vi "Display Raw Data.vi"(6 "Display":T2=enum."Channel B", 7 "Enum":T1, 8 "Data Format":T3, 9 "Processed B-Scan":sgl[][](array[numeric]), 10 "Length":i32, 11 "Raw Data In":u16[](array[numeric])) -> ()   [LabVIEW 2014]
uses:
  Type Defs/OCT DAQ Channel Data Type.ctl
  Type Defs/Display States.ctl
  Display Raw Data states.ctl
panel:
  out "Raw Data":u16[](graph)
  out "FFT Data":sgl[](graph)
  in  "Index":i32
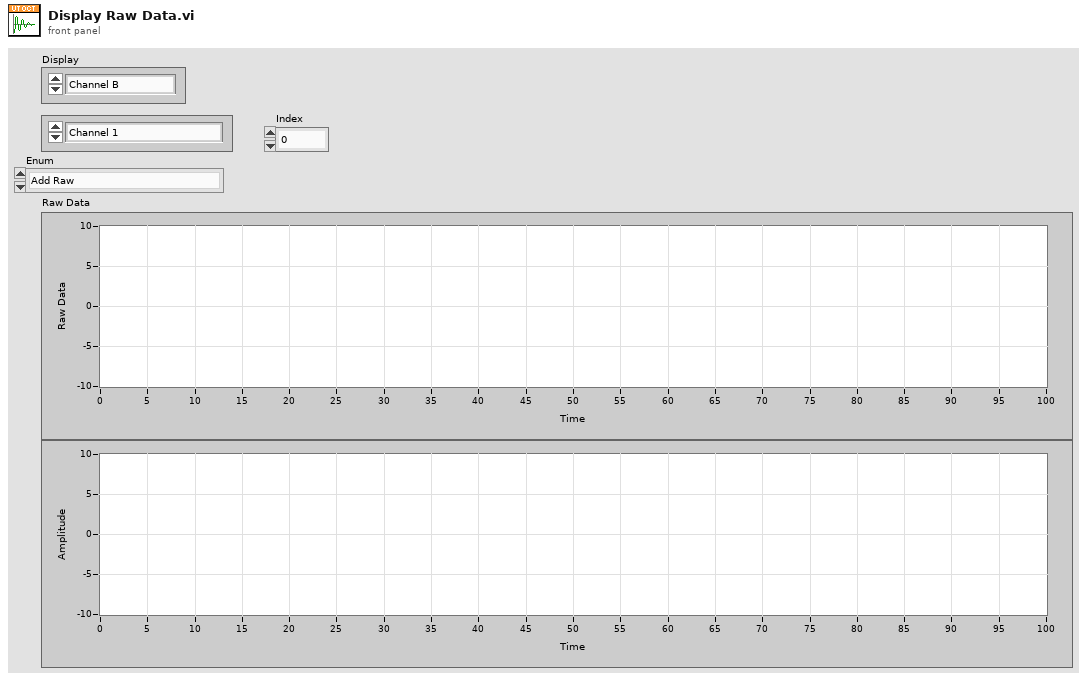
[diagram p1: front panel]
types:
  T1 = typedef "Display Raw Data states.ctl" = enum16{"Add Raw", "Add Processed", "Show"}
  T2 = typedef "Display States.ctl" = enum16{"Channel A", "Channel B"}
  T3 = typedef "OCT DAQ Channel Data Type.ctl" = enum16{"Channel 1", "Channel 2", "Channel 1 and 2"}
  T4 = enum32{"Invalid", "Standard", "Closed", "Hidden", "Minimized", "Maximized"}
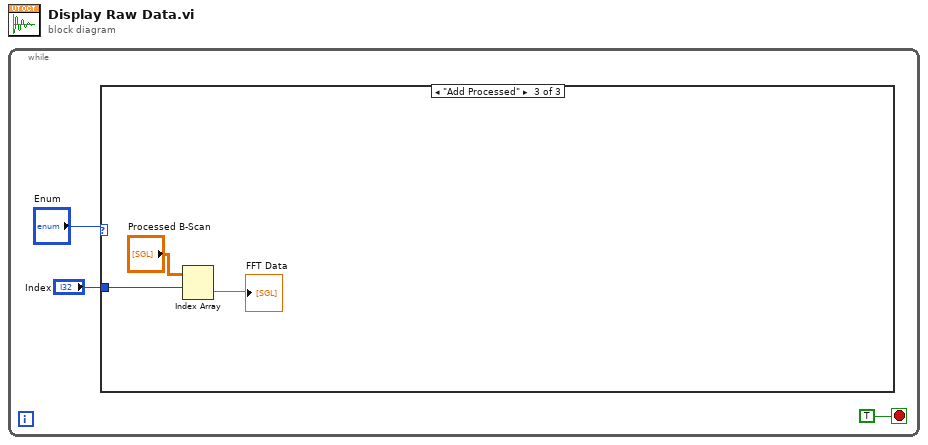
[diagram p0: block diagram]
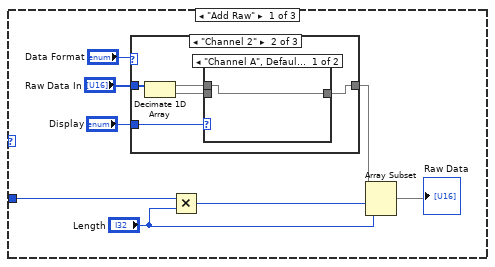
[diagram p2: hidden frame]
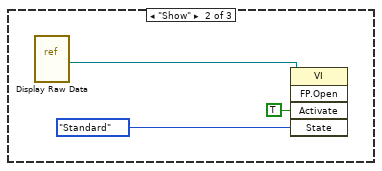
[diagram p6: hidden frame]
diagram:
  n1 = while {
    stop <- TRUE stop-if-true
    n2 = case shown="\"Add Processed\"" "Enum" {
      tunnel: "Index" -> [w5 _ w26]
      frame "Add Raw" {
        n3 = case shown="\"Channel 2\"" "Data Format" {
          tunnel: [w12 w15 w20] -> w8
          tunnel: "Raw Data In" -> [w12 w17 w20]
          tunnel: "Display" -> [_ w16 _]
          frame "Channel 1", Default {
          }
          frame "Channel 2" {
            n4 = Decimate 1D Array(w17) -> (w13:u16[], w14:u16[])
            n5 = case shown="\"Channel A\", Default" w16 {
              tunnel: [w18 w19] -> w15
              tunnel: w14 -> [_ w19]
              tunnel: w13 -> [w18 _]
              frame "Channel A", Default {
              }
              frame "Channel B" {
              }
            }
          }
          frame "Channel 1 and 2" {
          }
        }
        n6 = Multiply(x=w5, y="Length") -> (x*y=w11:i32)
        n7 = Array Subset(array=w8, index=w11, length="Length") -> (→"Raw Data":u16[])
      }
      frame "Show" {
        n8 = vi-ref "Display Raw Data.vi"() -> (w23:refnum<vi>)
        n9 = invoke class="VI" method="FP.Open"(reference=w23, "Activate"=TRUE ("Activate?"), "State"=T4."Standard") -> ()  [unwired: 2 in, 5 out]
      }
      frame "Add Processed" {
        n10 = Index Array(array="Processed B-Scan", index (row)=w26) -> (element=→"FFT Data":sgl[])  [unwired: 1 in]
      }
    }
  }
